vi "VISA BAR3 Write U8 vs U64.vi"() -> ()   [LabVIEW 2016]
uses:
  <vilib>/Platform/TimedLoop/XDataNode/timing_clust.ctl
  <vilib>/Platform/TimedLoop/XDataNode/nitl_modes.ctl
  <vilib>/Platform/TimedLoop/XDataNode/wakeup.ctl
  Source/GE 5565PIORC/GE 5565PIORC.lvclass/GE 5565PIORC.ctl
  <vilib>/Instr/_visa.llb/VISA Register Access Address Space.ctl
  Source/GE 5565PIORC/VIs/Registers/Local Configuration.LAS1RR.Address Range.Get.vi
  Source/GE 5565PIORC/VIs/Registers/Local Configuration.Get Register Offset.vi
  Source/GE 5565PIORC/GE 5565PIORC.lvclass
  <vilib>/platform/TimedLoop/XDataNode/XDataNode.xnode
  <vilib>/Platform/TimedLoop/XDataNode/XDNodeRunTimeDep.lvlib
panel:
  out "U64 Duration":dbl
  in  "U64s":i32=100
  out "U8 Duration":dbl
  in  "VISA resource name":refnum<visa-resource-name>
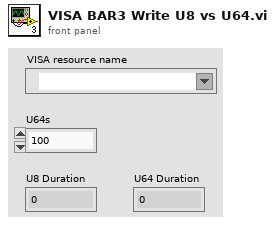
[diagram p1: front panel]
types:
  T1 = typedef "XDNodeRunTimeDep.lvlib/timing_clust.ctl" = cluster{"Expected End [f-1]":u64, "Actual End [f-1]":u64, "Finished Late? [f-1]":bool, "Expected End [i-1]":u64, "Actual End [i-1]":u64, "Finished Late? [i-1]":bool, "Expected Start [i]":u64, "Actual Start [i]":u64, "Expected Start [f]":u64, "Actual Start [f]":u64, "Source Name":string, "Structure Name":string, "Period":i64, "Deadline":i64, "Offset":i64, "Start":i64, "Priority":i32, "Timeout":i32, "Mode":T2, "Wakeup Reason":T3, "Error":errorcluster, "Source Type":string, "Secondary Source Type":string, "Global End Time":u64, "Global Start Time":u64, "Frame Duration":u64, "Iteration Duration":u64, "Assigned CPU":i32, "I/O Scan Engine Mode":u32}
  T2 = typedef "XDNodeRunTimeDep.lvlib/nitl_modes.ctl" = enum32{"No Change", "Process missed periods, maintain original phase", "Discard missed periods, maintain original phase", "Process missed periods, ignore original phase", "Discard missed periods, ignore original phase"}
  T3 = typedef "XDNodeRunTimeDep.lvlib/wakeup.ctl" = enum32{"Normal", "Aborted", "Asynchronous wakeup", "Timing source error", "Timed loop error", "Timeout"}
  T4 = typedef "VISA Register Access Address Space.ctl" = u16
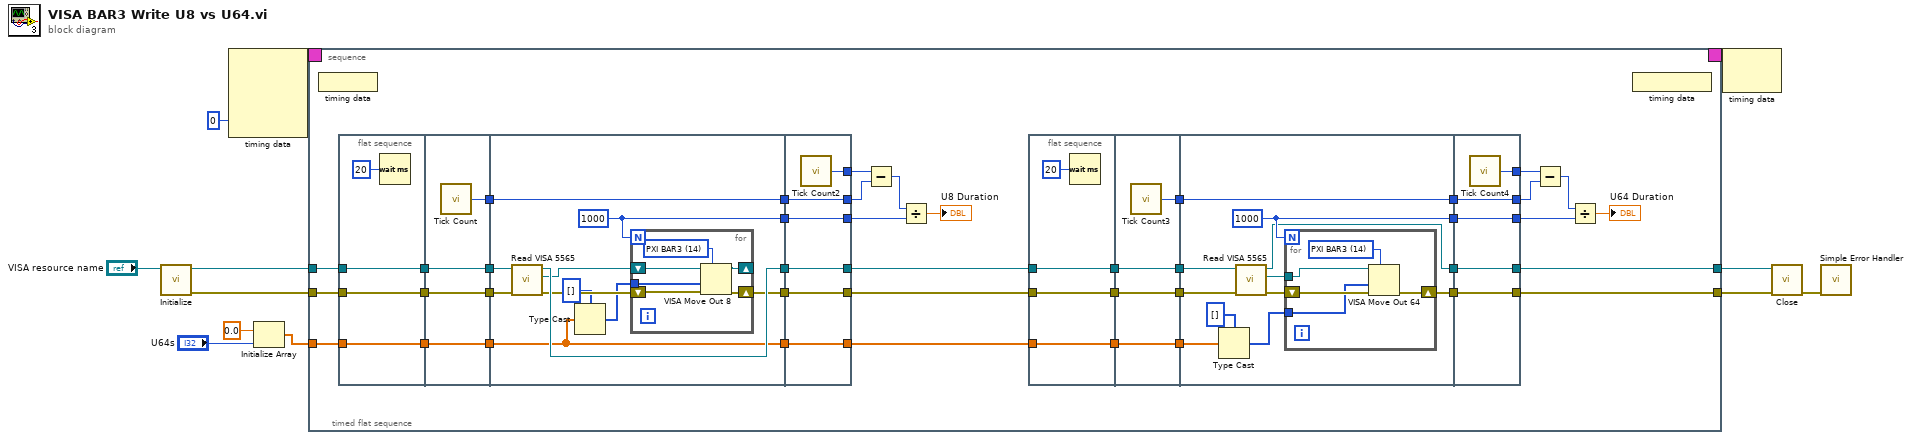
[diagram p0: block diagram]
diagram:
  n1 = call "Initialize.vi"("VISA resource name"="VISA resource name") -> ("error out"=w6:errorcluster, "GE 5565PIORC"=w7:refnum<class "GE 5565PIORC.lvclass">)  [unwired: 9 in]
  n2 = node-c288(0 ("Processor")) -> (w10:T1)  [unwired: 3 in]
  n3 = Initialize Array(0.0 ("element"), "U64s") -> (w1:dbl[])
  n4 = timed-sequence {
    timing: w10 -> [_]
    timing-out: [_] -> w9
    tunnel: w7 -> [w17]
    tunnel: w6 -> [w16]
    tunnel: [w14] -> w5
    tunnel: [w13] -> w4
    tunnel: w1 -> [w15]
    n5 = timed-flat-sequence {
      tunnel: w17 -> [w54]
      tunnel: w16 -> [w53]
      tunnel: w15 -> [w42]
      tunnel: [w22] -> w14
      tunnel: [w21] -> w13
      n6 = node-c288() -> ()  [unwired: 1 in]
      n7 = flat-sequence {
        tunnel: w54 -> [w90]
        tunnel: w53 -> [w89]
        tunnel: [w90] -> w51
        tunnel: [w89] -> w49
        tunnel: w42 -> [w88]
        tunnel: [w88] -> w40
        tunnel: [w95] -> w58
        tunnel: [w94] -> w52
        tunnel: w51 -> [w94]
        tunnel: [w93] -> w50
        tunnel: w49 -> [w93]
        tunnel: [w92] -> w41
        tunnel: w40 -> [w92]
        tunnel: w58 -> [w106]
        tunnel: [w106] -> w57
        tunnel: w52 -> [w105]
        tunnel: w50 -> [w100]
        tunnel: [w104] -> w48
        tunnel: [w103] -> w47
        tunnel: [w102] -> w46
        tunnel: w41 -> [w98]
        tunnel: [w98] -> w20
        tunnel: [w118] -> w56
        tunnel: [w117] -> w55
        tunnel: w57 -> [w117]
        tunnel: w48 -> [w116]
        tunnel: w47 -> [w115]
        tunnel: [w116] -> w24
        tunnel: [w115] -> w23
        tunnel: w46 -> [w114]
        tunnel: [w114] -> w44
        tunnel: w20 -> [w113]
        tunnel: [w113] -> w19
        frame #0 {
          n8 = Wait (ms)(milliseconds to wait=u32 20) -> ()  [unwired: 1 out]
        }
        frame #1 {
          n9 = call "Tick Count"() -> ("Tick Count(uSec)"=w95:u32)
        }
        frame #2 {
          w102 = 1000
          n10 = call "Read VISA 5565.vi"("error in (no error)"=w100, "GE 5565PIORC in"=w105) -> ("error out"=w99:errorcluster, "VISA 5565"=w101:refnum<visa-resource-name>, "GE 5565PIORC out"=w104:refnum<class "GE 5565PIORC.lvclass">)  [unwired: 7 in]
          n11 = Type Cast(type=u8[] [], x=w98) -> (*(type *) &x=w96:u8[])
          n12 = for {
            N: w102 -> [_]
            shift-right: [w110] -> _
            shift-left: w101 -> [w111]
            shift-right: [w109] -> w103
            shift-left: w99 -> [w108]
            tunnel: w96 -> [w107]
            w112 = T4 14 items=["VXI/VME A16"=1, "VXI/VME A24"=2, "VXI/VME A32"=3, "VXI/VME A64"=4, "PXI Memory Allocations"=9, "PXI Configuration"=10, "PXI BAR0"=11, "PXI BAR1"=12, "PXI BAR2"=13, "PXI BAR3"=14, "PXI BAR4"=15, "PXI BAR5"=16] ("Address Space")
            n13 = VISA Move Out 8(7:w112, 8:w108, 9:w107, 11:w111) -> (0:w109:errorcluster, 3:w110:refnum<visa-resource-name>)  [unwired: 1 in]
          }
        }
        frame #3 {
          n14 = call "Tick Count2"() -> ("Tick Count(uSec)"=w118:u32)
        }
      }
      n15 = Subtract(x=w56, y=w55) -> (x-y=w45:u32)
      n16 = Divide(x=w45, y=w44) -> (x/y=→"U8 Duration":dbl)
      n17 = flat-sequence {
        tunnel: w24 -> [w61]
        tunnel: w23 -> [w60]
        tunnel: [w61] -> w39
        tunnel: [w60] -> w38
        tunnel: w19 -> [w59]
        tunnel: [w59] -> w37
        tunnel: [w66] -> w36
        tunnel: [w65] -> w35
        tunnel: w39 -> [w65]
        tunnel: [w64] -> w34
        tunnel: w38 -> [w64]
        tunnel: [w63] -> w33
        tunnel: w37 -> [w63]
        tunnel: w36 -> [w77]
        tunnel: [w77] -> w32
        tunnel: w35 -> [w74]
        tunnel: w34 -> [w73]
        tunnel: [w76] -> w31
        tunnel: [w75] -> w30
        tunnel: w33 -> [w68]
        tunnel: [w70] -> w18
        tunnel: [w87] -> w29
        tunnel: [w86] -> w28
        tunnel: w32 -> [w86]
        tunnel: w31 -> [w85]
        tunnel: [w83] -> w22
        tunnel: [w85] -> w21
        tunnel: w30 -> [w84]
        tunnel: [w84] -> w26
        tunnel: w18 -> [w83]
        frame #0 {
          n18 = Wait (ms)(milliseconds to wait=u32 20) -> ()  [unwired: 1 out]
        }
        frame #1 {
          n19 = call "Tick Count3"() -> ("Tick Count(uSec)"=w66:u32)
        }
        frame #2 {
          w75 = 1000
          n20 = Type Cast(type=u64[] [], x=w68) -> (*(type *) &x=w67:u64[])
          n21 = call "Read VISA 5565.vi"("error in (no error)"=w73, "GE 5565PIORC in"=w74) -> ("error out"=w72:errorcluster, "VISA 5565"=w71:refnum<visa-resource-name>, "GE 5565PIORC out"=w70:refnum<class "GE 5565PIORC.lvclass">)  [unwired: 7 in]
          n22 = for {
            N: w75 -> [_]
            shift-right: [w81] -> w76
            shift-left: w72 -> [w82]
            tunnel: w71 -> [w79]
            tunnel: w67 -> [w78]
            w80 = T4 14 items=["VXI/VME A16"=1, "VXI/VME A24"=2, "VXI/VME A32"=3, "VXI/VME A64"=4, "PXI Memory Allocations"=9, "PXI Configuration"=10, "PXI BAR0"=11, "PXI BAR1"=12, "PXI BAR2"=13, "PXI BAR3"=14, "PXI BAR4"=15, "PXI BAR5"=16] ("Address Space")
            n23 = VISA Move Out 64(7:w80, 8:w82, 9:w78, 11:w79) -> (0:w81:errorcluster)  [unwired: 1 in, 1 out]
          }
        }
        frame #3 {
          n24 = call "Tick Count4"() -> ("Tick Count(uSec)"=w87:u32)
        }
      }
      n25 = Subtract(x=w29, y=w28) -> (x-y=w27:u32)
      n26 = Divide(x=w27, y=w26) -> (x/y=→"U64 Duration":dbl)
      n27 = node-c288() -> ()  [unwired: 1 out]
    }
  }
  n28 = node-c288(w9) -> ()  [unwired: 1 out]
  n29 = call "Close.vi"("error in (no error)"=w4, "GE 5565PIORC in"=w5) -> ("error out"=w11:errorcluster)  [unwired: 8 in, 1 out]
  n30 = call <vilib>:"Simple Error Handler.vi"("error in (no error)"=w11) -> ()  [unwired: 4 in, 5 out]
